vi "ReadFieldData.vi"(8 "error in (no error)":errorcluster, 10 "Index":i32, 11 "BME68x in":refnum<class "BME680.lvclass">) -> (0 "error out":errorcluster, 3 "BME68x out":refnum<class "BME680.lvclass">)   [LabVIEW 2022 SP3, in "BME680.lvlib" / "BME680.lvclass"]
uses:
  BME680.lvclass
  BME680.lvclass/BME680.ctl
  Typedefs/Data.ctl
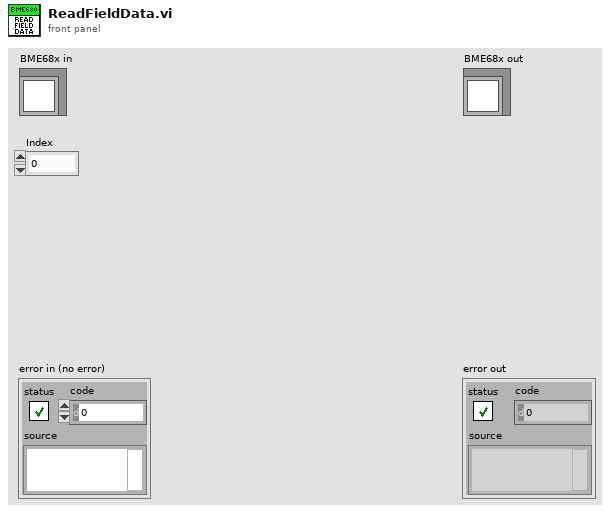
[diagram p1: front panel]
types:
  T1 = typedef "BME680.lvlib/BME680.lvclass/Data.ctl" = cluster{"Status":u8, "GasIdx":u8, "MeasIdx":u8, "ResHeat":u8, "iDac":u8, "GasWait":u8, "Temp":u16, "Pres":u32, "Hum":u8, "Gas Res":u8}
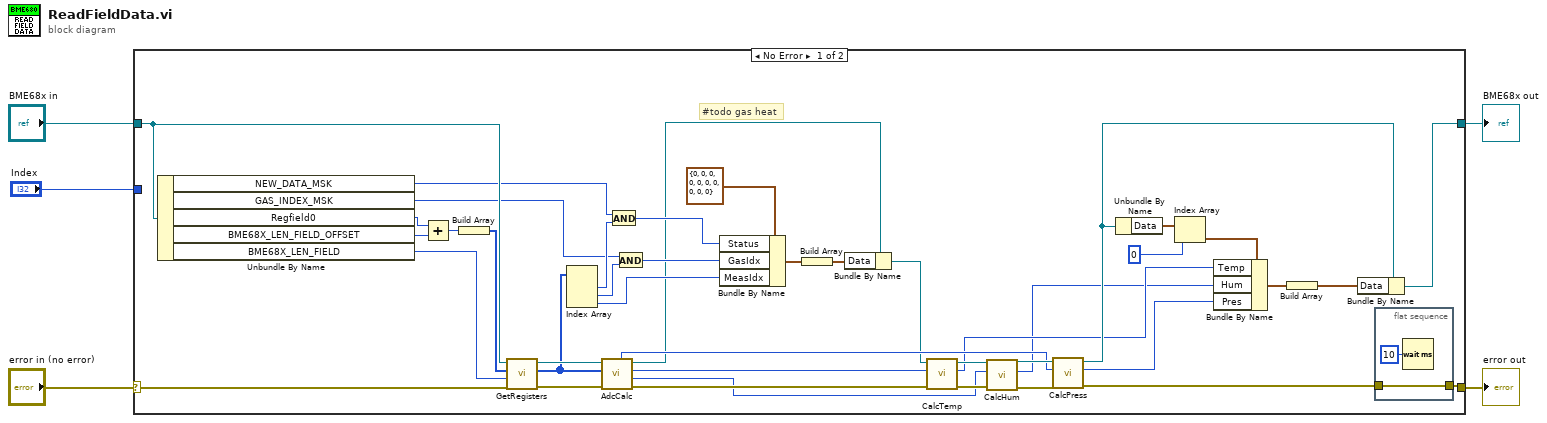
[diagram p0: block diagram]
diagram:
  n1 = case shown="No Error" "error in (no error)" {
    selector: "error in (no error)" -> [w47 w51]
    tunnel: [w24 w51] -> w4
    tunnel: [w15 w50] -> w2
    tunnel: "BME68x in" -> [w46 w50]
    tunnel: "Index" -> [_ _]
    frame No Error {
      # "#todo gas heat"
      n2 = Unbundle By Name(w46) -> ("NEW_DATA_MSK"=w39:u8, "GAS_INDEX_MSK"=w37:u8, "Regfield0"=w45:u8, "BME68X_LEN_FIELD_OFFSET"=w44:u8, "BME68X_LEN_FIELD"=w43:u8)
      n3 = Add(x=w45, y=w44) -> (x+y=w42:u8)
      n4 = Build Array(w42) -> (w41:u8[])
      n5 = call-dynamic "GetRegisters.vi"("error in (no error)"=w47, "Lenght"=w43, "Addr"=w41, "BME680 in"=w46) -> ("error out"=w34:errorcluster, "Data out"=w35:u8[], "BME680 out"=w36:refnum<class "BME680.lvclass">)  [unwired: 5 in]
      n6 = Index Array(array=w35) -> (element #1=w40:u8, element #2=w38:u8, element #3=w20:u8)  [unwired: 3 in]
      n7 = call "AdcCalc.vi"("error in (no error)"=w34, "Array"=w35, "BME680 in"=w36) -> ("error out"=w33:errorcluster, "Adc Hum"=w30:u32, "Adc Temp"=w32:u32, "BME680 out"=w19:refnum<class "BME680.lvclass">, "Adc Pres"=w26:u32)  [unwired: 4 in]
      n8 = And(x=w39, y=w40) -> (x .and. y?=w22:u8)
      n9 = And(x=w37, y=w38) -> (x .and. y?=w21:u8)
      n10 = Bundle By Name(cluster=T1 {"Status"=0, "GasIdx"=0, "MeasIdx"=0, "ResHeat"=0, "iDac"=0, "GasWait"=0, "Temp"=0, "Pres"=0, "Hum"=0, "Gas Res"=0} ("Data"), "Status"=w22, "GasIdx"=w21, "MeasIdx"=w20) -> (w18:T1)
      n11 = Build Array(w18) -> (w17:T1[])
      n12 = Bundle By Name(cluster=w19, "Data"=w17) -> (w16:refnum<class "BME680.lvclass">)
      n13 = call "CalcTemp.vi"("error in (no error)"=w33, "Adc_temp"=w32, "BME68x in"=w16) -> ("error out"=w31:errorcluster, "Temp"=w10:i16, "BME68x out"=w29:refnum<class "BME680.lvclass">)  [unwired: 6 in]
      n14 = call "CalcHum.vi"("error in (no error)"=w31, "Adc_Hum"=w30, "BME68x in"=w29) -> ("error out"=w28:errorcluster, "Hum"=w9:i32, "BME68x out"=w27:refnum<class "BME680.lvclass">)  [unwired: 6 in]
      n15 = call "CalcPress.vi"("error in (no error)"=w28, "Adc_press"=w26, "BME68x in"=w27) -> ("error out"=w25:errorcluster, "Press"=w8:i32, "BME68x out"=w14:refnum<class "BME680.lvclass">)  [unwired: 6 in]
      n16 = Unbundle By Name(w14) -> ("Data"=w13:T1[])
      n17 = Index Array(array=w13, index=0) -> (element=w11:T1)
      n18 = Bundle By Name(cluster=w11, "Temp"=w10, "Hum"=w9, "Pres"=w8) -> (w7:T1)
      n19 = Build Array(w7) -> (w6:T1[])
      n20 = Bundle By Name(cluster=w14, "Data"=w6) -> (w15:refnum<class "BME680.lvclass">)
      n21 = flat-sequence {
        tunnel: w25 -> [w49]
        tunnel: [w49] -> w24
        frame #0 {
          n22 = Wait (ms)(milliseconds to wait=u32 10) -> ()  [unwired: 1 out]
        }
      }
    }
    frame Error {
    }
  }
  "error out" <- w4
  "BME68x out" <- w2
